vi "Get List Information.vi"(10 "DQMH List":string, 11 "Tree Map":T1) -> ()   [LabVIEW 2020]
uses:
  <vilib>/National Instruments/Tree Map/Tree Map Data.ctl
  <vilib>/National Instruments/Tree Map/Tree Map.lvlib
panel:
  out "Library name":string
  out "Name":string
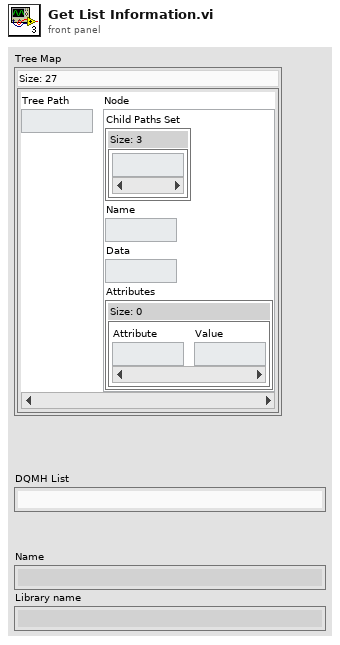
[diagram p1: front panel]
types:
  T1 = typedef "Tree Map.lvlib/Tree Map Data.ctl" = map{string, cluster{"Child Paths Set":set{string}, "Name":string, "Data":string, "Attributes":map{string, string}}}
  T2 = cluster{"Child Paths Set":set{string}, "Name":string, "Data":string, "Attributes":map{string, string}}
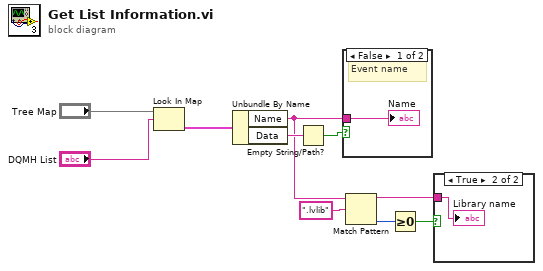
[diagram p0: block diagram]
diagram:
  n1 = Look In Map(map="Tree Map", key="DQMH List") -> (value=w8:T2)  [unwired: 1 in, 1 out]
  n2 = Unbundle By Name(w8) -> ("Name"=w5:string, "Data"=w7:string)
  n3 = Empty String/Path?(string/path=w7) -> (empty?=w6:bool)
  n4 = case shown="False" w6 {
    tunnel: w5 -> [w11 _]
    frame False {
      # "Event name"
      "Name" <- w11
    }
    frame True {
    }
  }
  n5 = Match Pattern(string=w5, regular expression=".lvlib") -> (before substring=w1:string, offset past match=w3:i32)  [unwired: 1 in, 2 out]
  n6 = Greater Or Equal To 0?(x=w3) -> (x >= 0?=w2:bool)
  n7 = case shown="True" w2 {
    tunnel: w1 -> [_ w12]
    frame False {
    }
    frame True {
      "Library name" <- w12
    }
  }
